vi "GUI.TestLauncher.vi"() -> ()   [LabVIEW 2022 SP3, in "GUI.lvclass"]
doc: "JKI State Machine Objects (SMO) 1.0.0.5\nJKI - JKI\nCopyright (c) 2016, JKI"
uses:
  GUI.lvclass
  <vilib>/JKI/JKI SMO/SMO/Typedefs/SMOState --Enum.ctl
  C:/Program Files (x86)/National Instruments/LabVIEW 2022/vi.lib/JKI/JKI SMO/SMO/SMO.lvclass
  Typedefs/Value.ctl
  <vilib>/JKI/JKI SMO/SMO/SMO.lvclass/SMO.ctl
  <vilib>/JKI/JKI SMO/SMO/Private/ReftoDVR--SMO.vi
  GUI.lvclass/GUI.ctl
  <vilib>/JKI/JKI SMO/SMO/SMO.lvclass
  C:/Program Files (x86)/National Instruments/LabVIEW 2022/vi.lib/JKI/JKI SMO/SMO.UI/SMO.UI.lvclass
  D:/DSUsers/uib01493/000_SD_Card/009_Projects/CIS_580/SReTT_GUI/002_SRC/GUI/GUI.lvclass
  <vilib>/JKI/JKI SMO/SMO.UI/SMO.UI.lvclass
panel:
  out "State":T1
  out "New Value Event":string
  in  "Send":bool
  in  "Value":string
  out "error out":errorcluster
  in  "Stop":bool
  # "Basic SMO byRef Test Launcher"
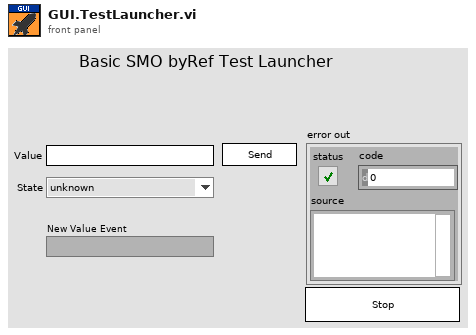
[diagram p1: front panel]
types:
  T1 = typedef "SMO.lvclass/SMOState --Enum.ctl" = enum16{"unknown", "Created", "Started", "Stopped"}
  T2 = typedef "GUI.lvclass/Value.ctl" = string
  T3 = typedef "GUI.lvclass/PublicEvents--Cluster.ctl" = cluster{"Value Changed":refnum<user-event>}
  T4 = typedef "SMO.lvclass/Public Events.ctl" = cluster{"Error":refnum<user-event>, "State":refnum<user-event>, "Reserve State":refnum<user-event>}
  T5 = cluster{"Event Registration Refnum":refnum<event-registration>}
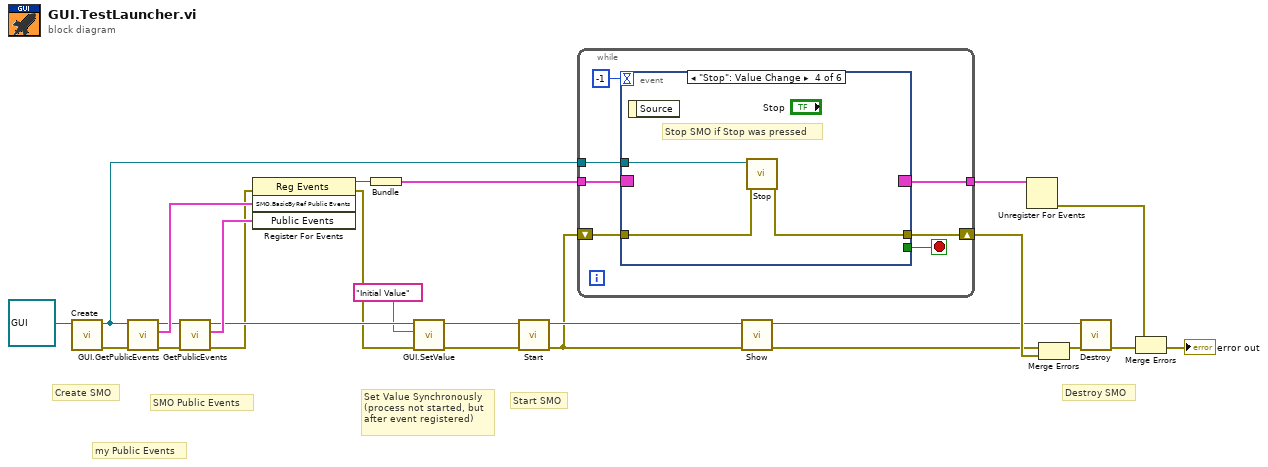
[diagram p0: block diagram]
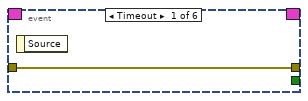
[diagram p2: hidden frame]
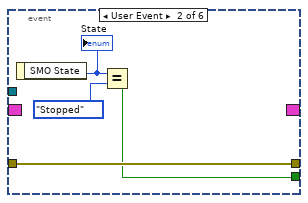
[diagram p3: hidden frame]
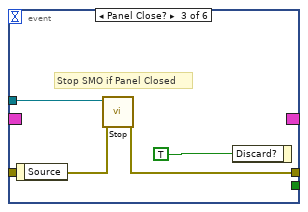
[diagram p4: hidden frame]
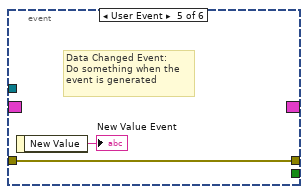
[diagram p5: hidden frame]
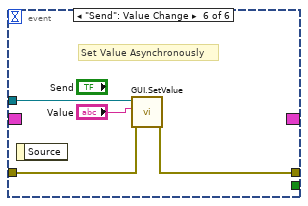
[diagram p6: hidden frame]
diagram:
  # "Set Value Synchronously\n(process not started, but\nafter event registered)"
  # "SMO Public Events"
  # "my Public Events"
  # "Start SMO"
  # "Destroy SMO"
  # "Create SMO"
  n1 = call <vilib>:"Create.vi"("SMO"=refnum<class "GUI.lvclass"> refnum ("SMO.Template.lvclass")) -> ("error out"=w18:errorcluster, "SMO out"=w15:refnum<class "GUI.lvclass">)  [unwired: 8 in, 1 out]
  n2 = call "GUI.GetPublicEvents.vi"("error in (no error)"=w18, "GUI"=w15) -> ("error out"=w13:errorcluster, "SMO.BasicByRef Public Events"=w17:T3, "GUI out"=w14:refnum<class "GUI.lvclass">)  [unwired: 7 in]
  n3 = call <vilib>:"GetPublicEvents.vi"("error in (no error)"=w13, "SMO"=w14) -> ("error out"=w7:errorcluster, "Public Events"=w12:T4, "SMO out"=w11:refnum<class "GUI.lvclass">)  [unwired: 7 in]
  n4 = register-events(error in=w7, w17, w12) -> (reference out=w16:refnum<event-registration>, error out=w6:errorcluster)  [unwired: 1 in]
  n5 = Bundle("Event Registration Refnum"=w16) -> (w24:T5)  [unwired: 1 in]
  n6 = call "GUI.SetValue.vi"("error in (no error)"=w6, "Value"=T2 "Initial Value", "GUI"=w11) -> ("error out"=w9:errorcluster, "GUI out"=w10:refnum<class "GUI.lvclass">)  [unwired: 6 in, 1 out]
  n7 = call <vilib>:"Start.vi"("error in (no error)"=w9, "SMO"=w10) -> ("error out"=w1:errorcluster, "SMO out"=w4:refnum<class "GUI.lvclass">)  [unwired: 8 in]
  n8 = while {
    shift-right: [w31] -> w23
    shift-left: w1 -> [w30]
    tunnel: w24 -> [w29]
    tunnel: [w28] -> w25
    tunnel: w15 -> [w27]
    stop <- w32 stop-if-true
    n9 = event shown="[3] \"Stop\": Value Change" {
      selector: w29 -> [_ _ _ _ _ _]
      dyn-events: [_ _ _ _ _ _] -> w28
      timeout: -1 -> [_ _ _ _ _ _]
      tunnel: [_ w34 _ _ _ _] -> w32
      tunnel: w27 -> [_ _ w41 w44 _ w50]
      tunnel: [w33 w37 w40 w43 w46 w47] -> w31
      tunnel: w30 -> [w33 w37 w39 w42 w46 w48]
      event Timeout {
        n10 = event-data() -> ()  [unwired: 1 in, 1 out]
      }
      event User Event {
        n11 = event-data() -> ("SMO State"=w36:T1)  [unwired: 1 in]
        "State" <- w36
        n12 = Equal?(x=w36, y=SMOState_--Enum."Stopped") -> (x = y?=w34:bool)
      }
      event Panel Close? {
        # "Stop SMO if Panel Closed"
        n13 = event-data() -> ()  [unwired: 1 in, 1 out]
        n14 = call <vilib>:"Stop.vi"("error in (no error)"=w39, "SMO"=w41) -> ("error out"=w40:errorcluster)  [unwired: 8 in, 1 out]
        n15 = event-data("Discard?"=TRUE ("OK")) -> ()  [unwired: 1 in, 1 out]
      }
      event "Stop": Value Change {
        # "Stop SMO if Stop was pressed"
        n16 = event-data() -> ()  [unwired: 1 in, 1 out]
        n17 = call <vilib>:"Stop.vi"("error in (no error)"=w42, "SMO"=w44) -> ("error out"=w43:errorcluster)  [unwired: 8 in, 1 out]
      }
      event User Event {
        # "Data Changed Event:\nDo something when the\nevent is generated"
        n18 = event-data() -> ("New Value"=→"New Value Event":string)  [unwired: 1 in]
      }
      event "Send": Value Change {
        # "Set Value Asynchronously"
        n19 = event-data() -> ()  [unwired: 1 in, 1 out]
        n20 = call "GUI.SetValue.vi"("error in (no error)"=w48, "Value"="Value", "GUI"=w50) -> ("error out"=w47:errorcluster)  [unwired: 6 in, 2 out]
      }
    }
  }
  n21 = call <vilib>:"Show.vi"("error in (no error)"=w1, "SMO.UI"=w4) -> ("error out"=w2:errorcluster, "SMO.UI out"=w3:refnum<class "GUI.lvclass">)  [unwired: 8 in]
  n22 = Unregister For Events(event registration refnum=w25) -> (error out=w22:errorcluster)  [unwired: 1 in]
  n23 = Merge Errors(w2, w23) -> (w5:errorcluster)
  n24 = call <vilib>:"Destroy.vi"("error in (no error)"=w5, "SMO"=w3) -> ("error out"=w20:errorcluster)  [unwired: 9 in]
  n25 = Merge Errors(w22, w20) -> (→"error out":errorcluster)
